vi "Set Thermocouple Meas Mode.vi"(8 "error in (no error)":errorcluster, 10 "Temperature Units (22: Temperature in degrees Celsius)":u32(ring)=22 items=["Unitless", "Frequency in units of hertz", "Frequency in units of kilohertz", "Frequency in units of megahertz", "Volts in units of microvolts", "Volts in units of millivolts", "Volts in units of volts", "Volts in units of kilovolts", "Current in units of microamperes", "Current in units of milliamps", "Current in units of amps", "Percent", "Parts-per-million", "Volts in units of decibels referenced to 1 milliwatt into 600 W load", "Resistance in units of ohms", "Resistance in units of kilohms", "Resistance in units of megohms", "Capacitance in units of nanofarads", "Capacitance in units of picofarads", "Capacitance in units of  microfarads", "Capacitance in units of millifarads", "Capacitance in units of farads", "Temperature in degrees Celsius", "Temperature in degrees Fahrenheit", "Period in units of nanoseconds", "Period in units of microseconds", "Period in units of milliseconds", "Period in units of seconds", "Pound-force pre square inch", "Meters of mercury", "Inches of mercury", "Inches of water", "Feet of water", "Meters of water", "Bar", "Pascal", "Grams per centimeter squared", "Inches of water @ 60 degrees Farhenheit", "Decibels"], 11 "VISA resource name":refnum<visa-resource-name>) -> (0 "error out":errorcluster, 3 "VISA resource name out":refnum<visa-resource-name>)   [LabVIEW 2014, in "Fluke 5XXX Series Multicalibrators.lvlib"]
doc: "This VI selects mode to measure the thermocouple temperature that is attached to the Calibrator TC terminals.\n\nNote:\n\nThis VI is available only for instrument models 5500A and 5520A."
uses:
  Fluke 5XXX Series Multicalibrators.lvlib
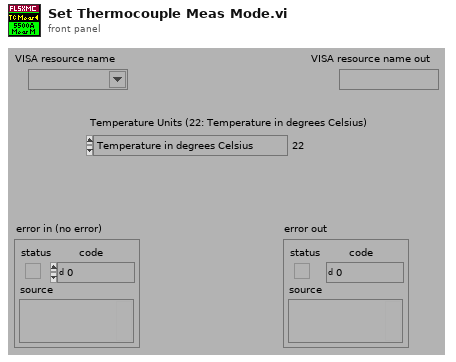
[diagram p1: front panel]
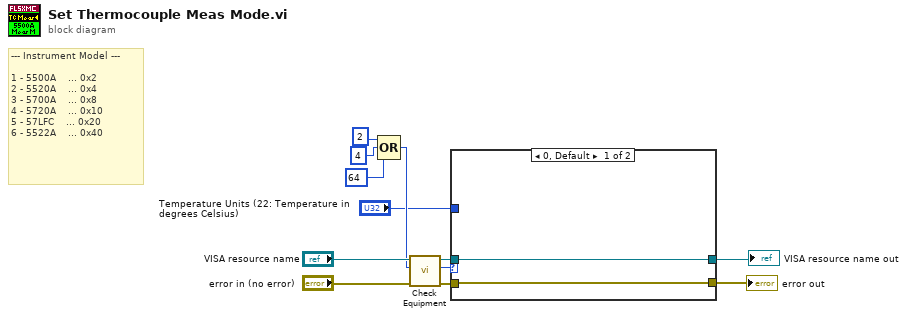
[diagram p0: block diagram]
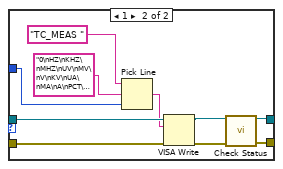
[diagram p2: hidden frame]
diagram:
  # "--- Instrument Model ---\n\n1 - 5500A    ... 0x2\n2 - 5520A    ... 0x4\n3 - 5700A    ... 0x8\n4 - 5720A    ... 0x10\n5 - 57LFC    ... 0x20\n6 - 5522A    ... 0x40"
  n1 = Compound Arithmetic op=OR(2 ("Numeric"), 4 ("Numeric"), 64 ("Numeric")) -> (w3:i32)
  n2 = call "Check Equipment.vi"("error in (no error)"="error in (no error)", "Bit Mask"=w3, "VISA resource name"="VISA resource name") -> ("error out"=w12:errorcluster, "Present?"=w11:u32, "VISA resource name out"=w10:refnum<visa-resource-name>)  [unwired: 6 in]
  n3 = case shown="0, Default" w11 {
    tunnel: [w13 w17] -> w6
    tunnel: w12 -> [w14 w23]
    tunnel: w10 -> [w13 w22]
    tunnel: [w14 w20] -> w7
    tunnel: "Temperature Units (22: Temperature in degrees Celsius)" -> [_ w16]
    frame 0, Default {
    }
    frame 1 {
      n4 = Pick Line(string ("")="TC_MEAS " ("Reset Command"), multi-line string="0\nHZ\nKHZ\nMHZ\nUV\nMV\nV\nKV\nUA\nMA\nA\nPCT\nPPM\nDBM\nOHM\nKOHM\nMOHM\nNF\nPF\nUF\nMF\nF\nCEL\nFAR\nNS\nUS\nMS\nS\nPSI\nMHG\nINHG\nINH2O\nFTH2O\nMH2O\nBAR\nPAL\nG/CM2\nINH2O60F\nDB", line index=w16) -> (output string=w21:string)
      n5 = VISA Write(VISA resource name=w22, write buffer=w21, error in (no error)=w23) -> (VISA resource name out=w18:refnum<visa-resource-name>, error out=w19:errorcluster)  [unwired: 1 out]
      n6 = call "Check Status.vi"("VISA resource name"=w18, "error in (no error)"=w19) -> ("VISA resource name out"=w17:refnum<visa-resource-name>, "error out"=w20:errorcluster)  [unwired: 12 in]
    }
  }
  "VISA resource name out" <- w6
  "error out" <- w7
